vi "Launch from TestStand.vi"(8 "error in":errorcluster, 11 "Run as Singleton? (F)":bool) -> (0 "error out":errorcluster, 3 "Module ID out":i32)   [LabVIEW 2022 SP3, in "Serial-Com-Module.lvlib"]
uses:
  Serial-Com-Module.lvlib
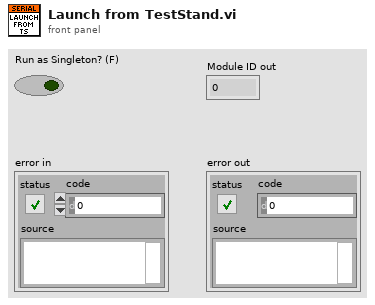
[diagram p1: front panel]
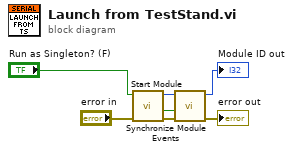
[diagram p0: block diagram]
diagram:
  n1 = call "Start Module.vi"("error in"="error in", "Run as Singleton? (F)"="Run as Singleton? (F)") -> ("error out"=w6:errorcluster, "Wait for Event Sync?"=w5:bool, "Module ID"=w7:i32)  [unwired: 6 in, 1 out]
  n2 = call "Synchronize Module Events.vi"("error in"=w6, "Wait for Event Sync?"=w5, "Module ID in"=w7) -> ("error out"=→"error out":errorcluster, "Module ID out"=→"Module ID out":i32)  [unwired: 7 in]
